vi "FPGA_Main.vi"() -> ()   [LabVIEW 2017]
uses:
  <vilib>/rvi/Emulation/niFpgaGetClockAttributes.vi
  <vilib>/rvi/Emulation/niFpgaSctlEmulationGetInTimedLoop.vi
  <vilib>/rvi/Emulation/niFpgaEmulationReportErrorSimple.vi
  <vilib>/rvi/eio/common/nirviEmuTemplateMethod_errors.vi
  <vilib>/rvi/Emulation/niFpgaCriticalErrorInLSC.vi
  <vilib>/eio/EIONode/EIONode.xnode
panel:
  out "Velocity Right (m/s)":sgl
  out "Raw ms Difference R":u32
  in  "Stop R":bool
  out "Velocity Left (m/s)":sgl
  out "Raw ms Difference L":u32
  in  "Stop L":bool
  out "BR Raw":bool
  out "BR Count":u8
  in  "Reset BR":bool
  out "BR Tape":bool
  out "FL Raw":bool
  out "FL Count":u8
  in  "Reset FL":bool
  out "BL Raw":bool
  out "BL Count":u8
  in  "Reset BL":bool
  out "BL Tape":bool
  out "FR Raw":bool
  out "FR Count":u8
  in  "Reset FR":bool
  out "Tick Count(uSec)":u32
  out "Right Velocity":sgl
  out "Left Velocity":sgl
  out "Right LS Fault":bool
  out "Left LS Fault":bool
  out "Right Tape Count":u32
  out "Left Tape Count":u32
  out "test time":u32
  out "PCS 4 Position":i16
  out "PCS 3 Position":i16
  out "PCS 2 Position":i16
  out "PCS 1 Position":i16
  out "Levitating?":bool
  out "Levitation Height":sgl format="%.14g"
  out "CJC Voltage":fxp<+/-,24,-2> format="%.26g"
  out "TC Voltages":fxp<+/-,25,-1>[](array[numeric]) format="%.26g"
  out "Reserve Battery Current":fxp<+/-,55,8>=25.777777883741592 format="%.14g"
  out "Primary Battery 2 Current":fxp<+/-,55,8>=25.777777883741592 format="%.14g"
  out "Primary Battery 1 Current":fxp<+/-,55,8>=25.777777883741592 format="%.14g"
  out "Reserve Battery Critical":bool
  out "Reserve Battery Low":bool
  out "Primary Battery 2 Critical":bool
  out "Primary Battery 2 Low":bool
  out "Primary Battery 1 Critical":bool
  out "Primary Battery 1 Low":bool
  out "Reserve Battery Voltage":sgl format="%.14g"
  out "Primary Battery 2 Voltage":sgl format="%.14g"
  out "Primary Battery 1 Voltage":sgl format="%.14g"
  out "Downstream 2 Pressure Fault":bool
  out "Ambient Pressure":sgl format="%.2f"
  out "Downstream Right Pressure":sgl format="%.2f"
  out "Tank Pressure":sgl format="%.2f"
  out "Downstream Left Pressure":sgl format="%.2f"
  out "Downstream Pressure Low":bool
  out "Tank Pressue Low":bool
  out "Downstream Pressure Fault":bool
  out "Tank Pressure Fault":bool
  out "Pusher Connected":bool
  out "IR Fault":bool
  out "IR 2 RAW":sgl format="%.21g"
  out "IR 1 RAW":sgl format="%.21g"
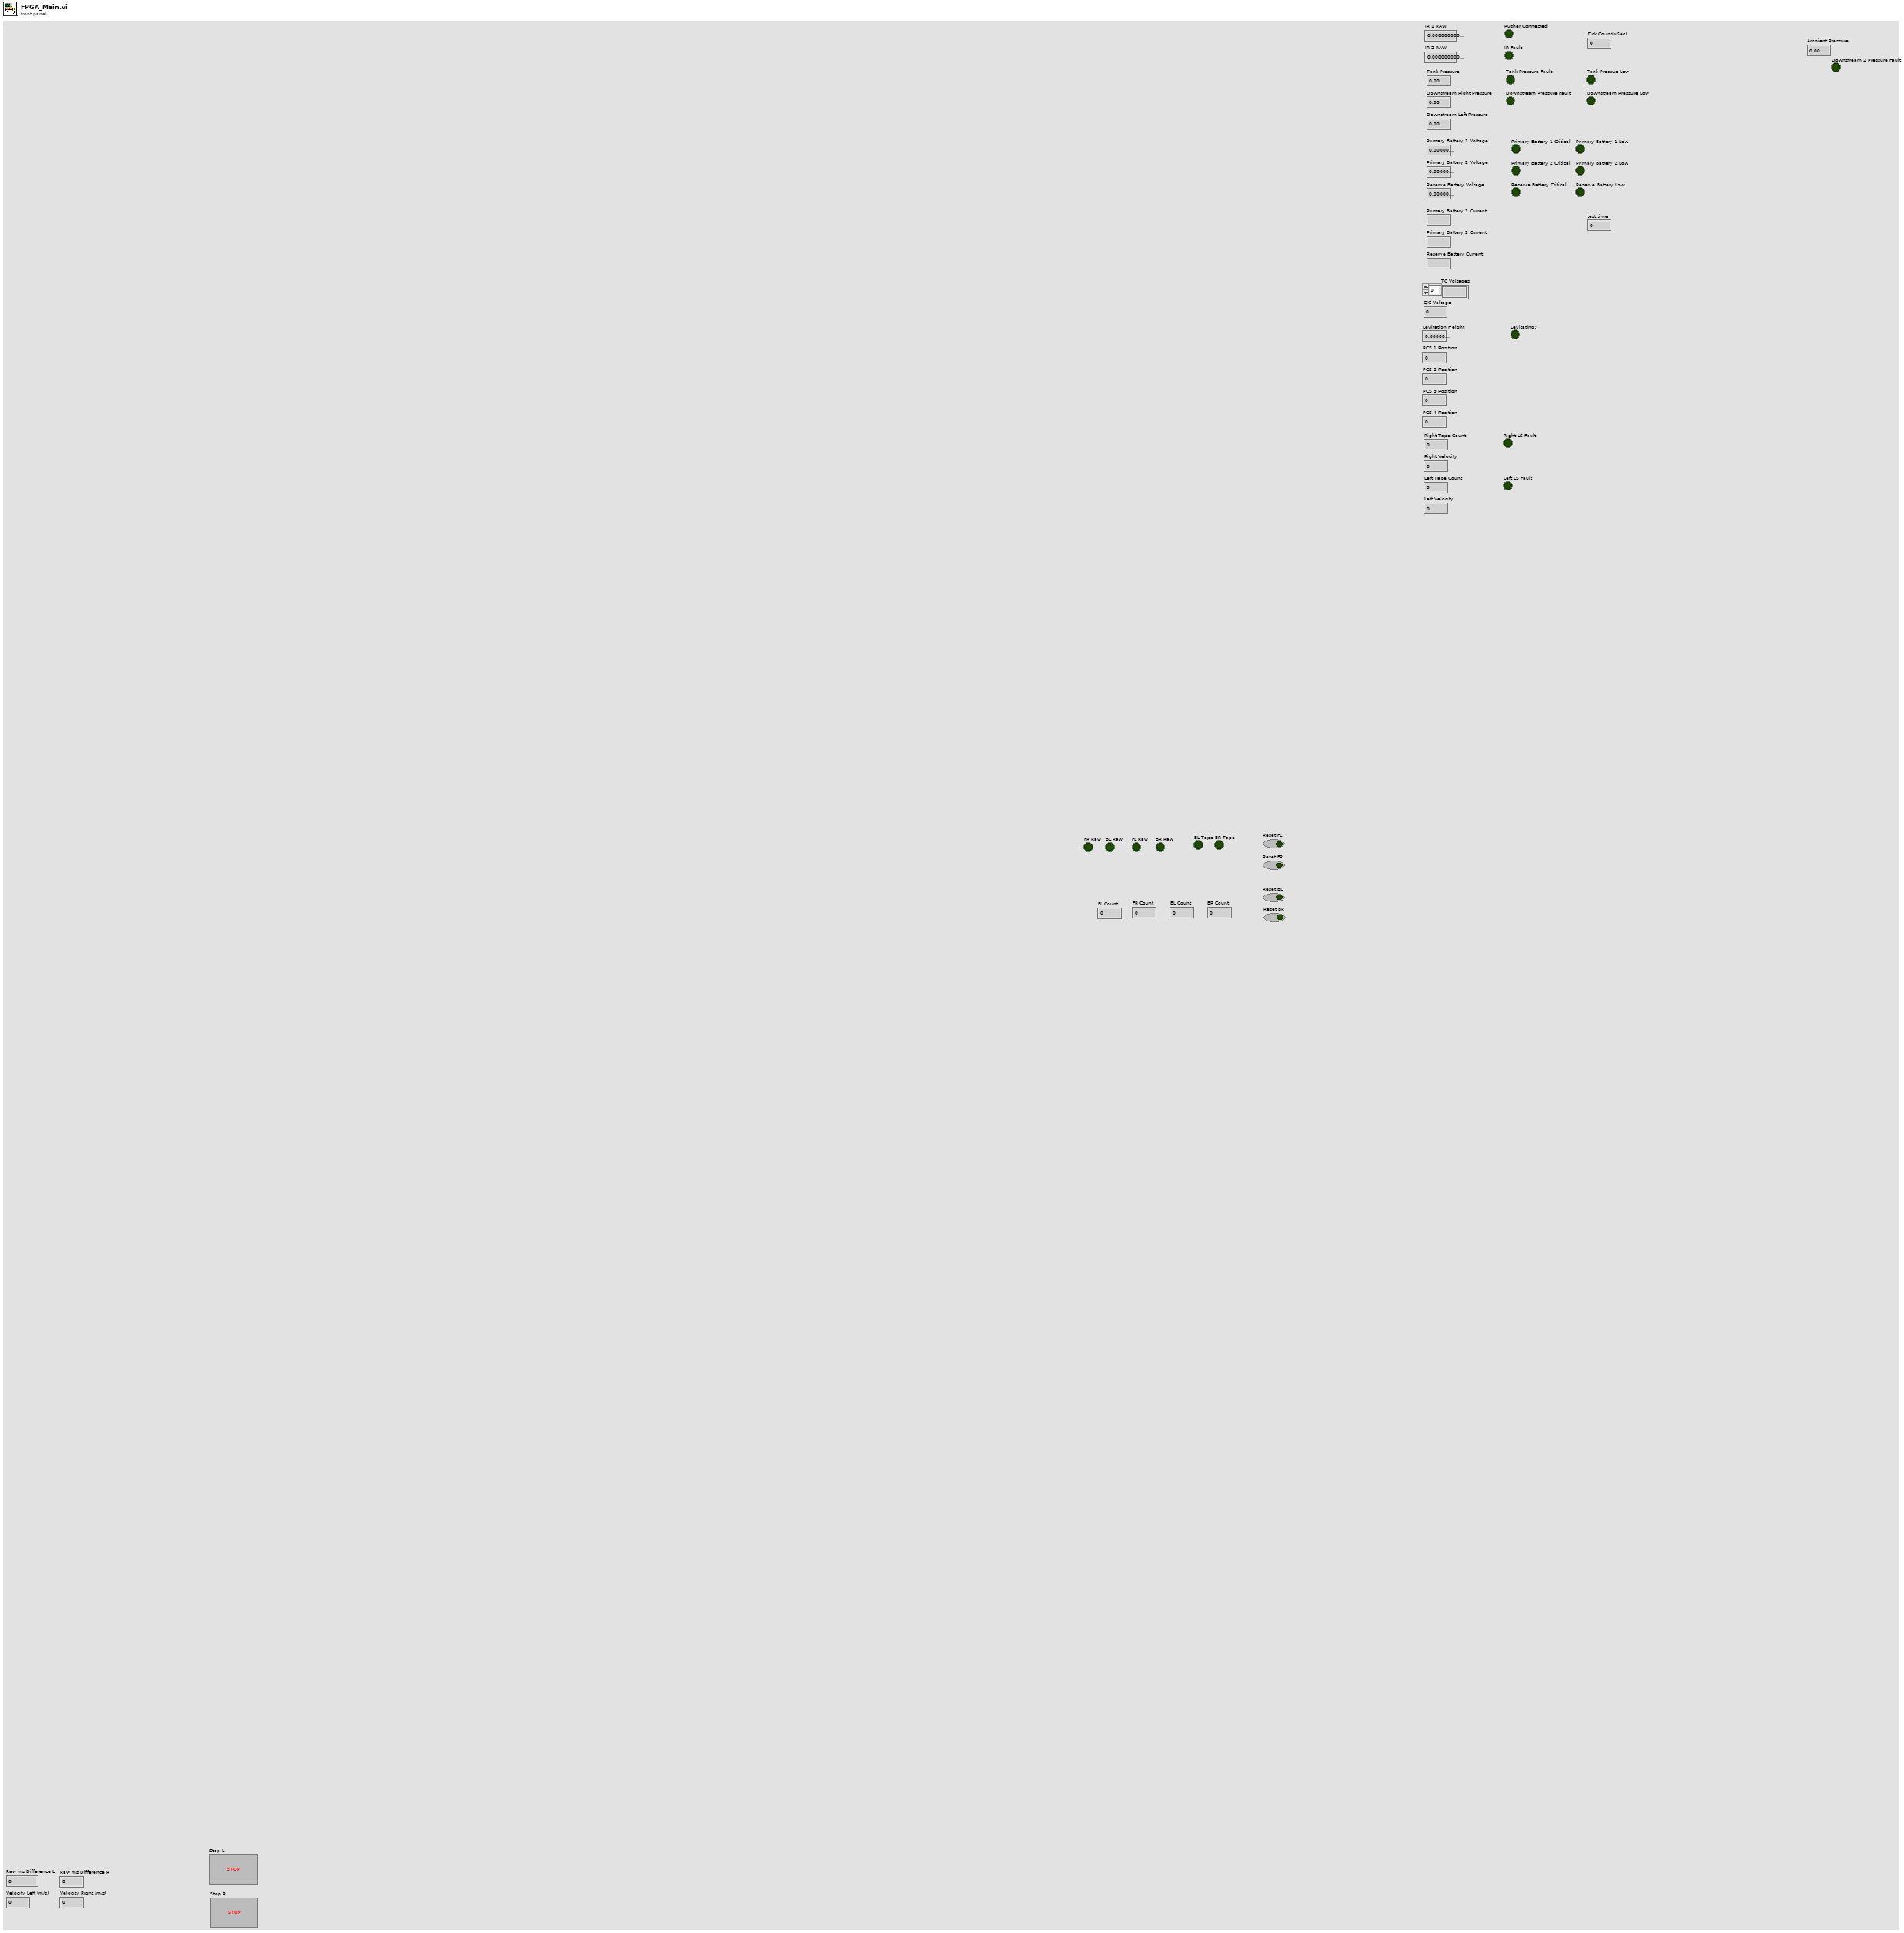
[diagram p1: front panel]
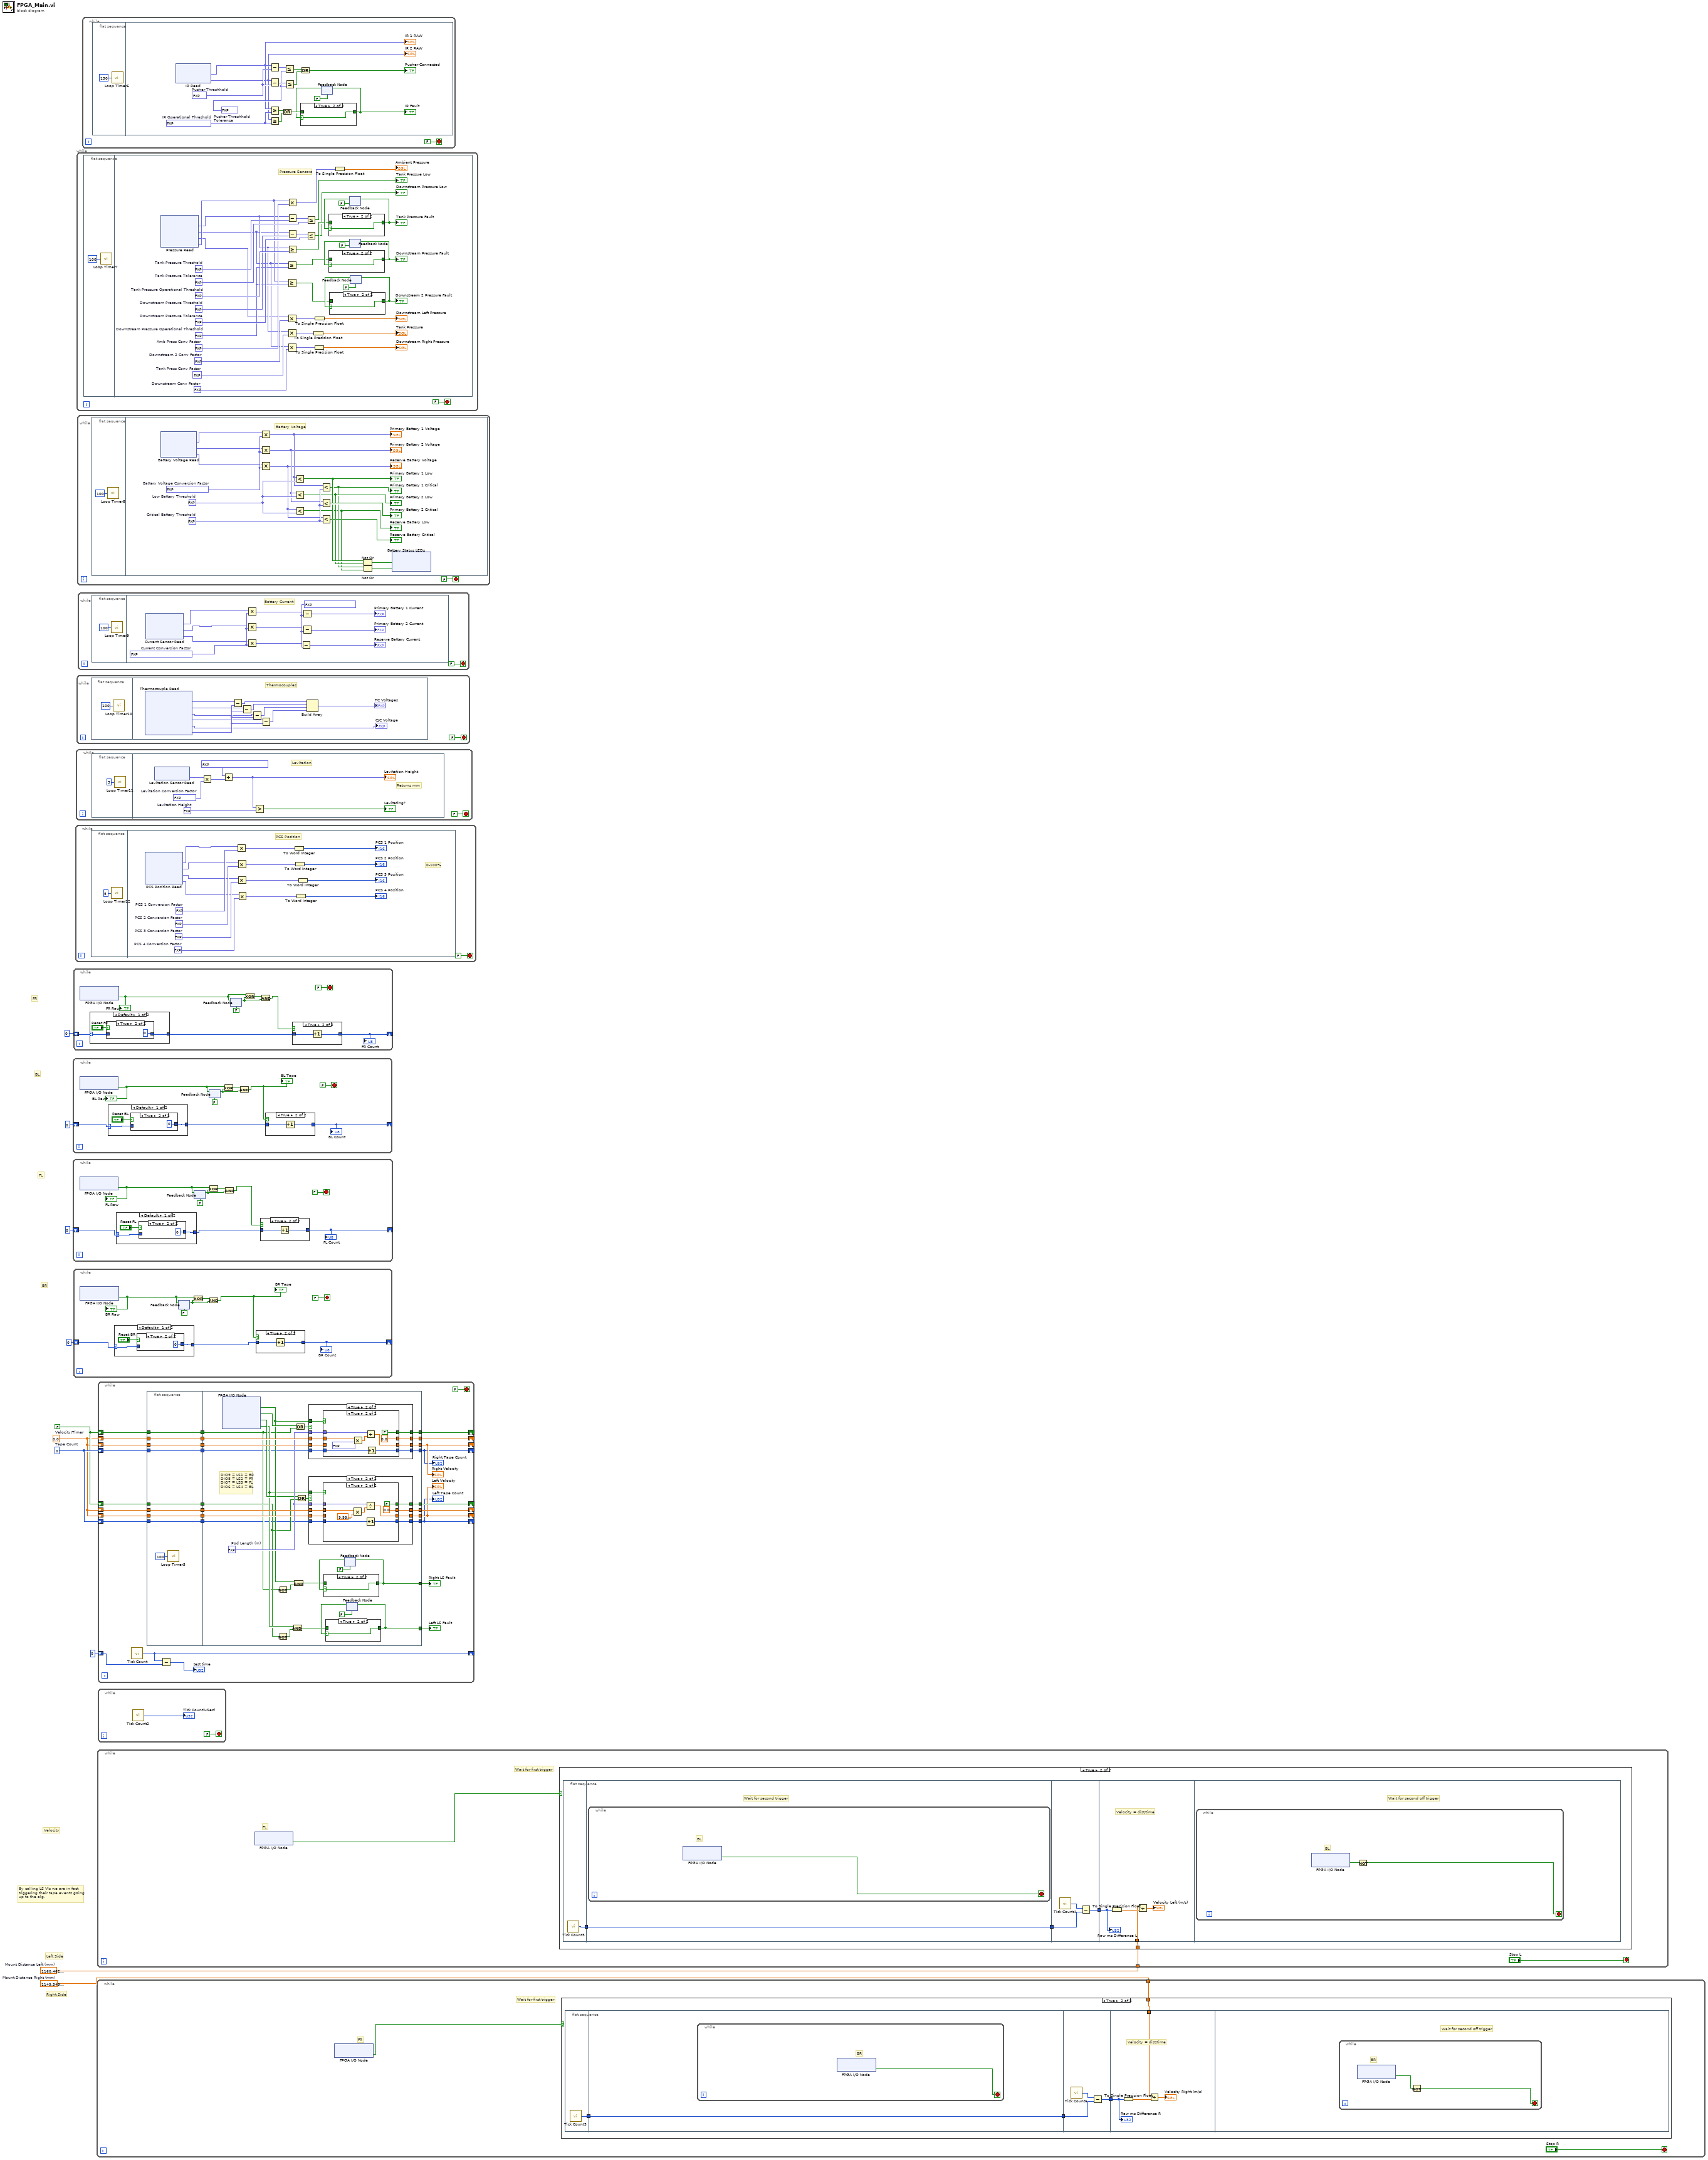
[diagram p0: block diagram]
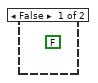
[diagram p2: hidden frame]
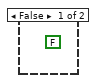
[diagram p3: hidden frame]
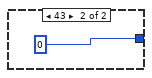
[diagram p5: hidden frame]
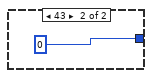
[diagram p8: hidden frame]
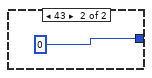
[diagram p11: hidden frame]
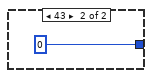
[diagram p14: hidden frame]
diagram:
  w1 = sgl 1149.35  # Mount Distance Right (mm)
  w2 = sgl 1160.4625  # Mount Distance Left (mm)
  w9 = FALSE
  w10 = u32 0  # Tape Count
  w7 = sgl 0.0  # Velocity/Timer
  # "Right Side"
  # "Left Side"
  # "By calling LS VIs we are in fact\ntriggering their tape events going\nup to the alg."
  # "Velocity"
  # "BR"
  # "FL"
  # "BL"
  # "FR"
  n1 = while {
    shift-right: [w14] -> _
    shift-left: u8 0 -> [w12]
    stop <- FALSE stop-if-true
    n2 = xnode "FPGA I/O Node"() -> ("Mod2/DIO8"=w15:bool)  [unwired: 1 in, 1 out]
    "BL Raw" <- w15
    n3 = case shown="Default" w12 {
      selector: w12 -> [w21 _]
      tunnel: [w20 u8 0] -> w11
      frame Default {
        n4 = case shown="True" "Reset BL" {
          tunnel: w21 -> [w23 _]
          tunnel: [w23 u8 0] -> w20
          frame False {
          }
          frame True {
          }
        }
      }
      frame 43 {
      }
    }
    n5 = feedback #1(FALSE ("Mod2/DIO2")) -> (w18:bool)
    n6 = feedback-in #1(w15) -> ()
    n7 = Exclusive Or(1:w18, 2:w15) -> (0:w17:bool)
    n8 = And(x=w17, y=w18) -> (x .and. y?=w13:bool)
    "BL Tape" <- w13
    n9 = case shown="True" w13 {
      tunnel: [w26 w28] -> w14
      tunnel: w11 -> [w26 w27]
      frame False {
      }
      frame True {
        n10 = Increment(x=w27) -> (x+1=w28:u8)
      }
    }
    "BL Count" <- w14
  }
  n11 = while {
    shift-right: [w31] -> _
    shift-left: u8 0 -> [w30]
    stop <- FALSE stop-if-true
    n12 = xnode "FPGA I/O Node"() -> ("Mod2/DIO7"=w33:bool)  [unwired: 1 in, 1 out]
    "FL Raw" <- w33
    n13 = case shown="Default" w30 {
      selector: w30 -> [w39 _]
      tunnel: [w38 u8 0] -> w29
      frame Default {
        n14 = case shown="True" "Reset FL" {
          tunnel: w39 -> [w41 _]
          tunnel: [w41 u8 0] -> w38
          frame False {
          }
          frame True {
          }
        }
      }
      frame 43 {
      }
    }
    n15 = feedback #2(FALSE ("Mod2/DIO2")) -> (w34:bool)
    n16 = feedback-in #2(w33) -> ()
    n17 = Exclusive Or(1:w34, 2:w33) -> (0:w35:bool)
    n18 = And(x=w35, y=w34) -> (x .and. y?=w32:bool)
    n19 = case shown="True" w32 {
      tunnel: [w44 w46] -> w31
      tunnel: w29 -> [w44 w45]
      frame False {
      }
      frame True {
        n20 = Increment(x=w45) -> (x+1=w46:u8)
      }
    }
    "FL Count" <- w31
  }
  n21 = while {
    shift-right: [w50] -> _
    shift-left: u8 0 -> [w48]
    stop <- FALSE stop-if-true
    n22 = xnode "FPGA I/O Node"() -> ("Mod2/DIO6"=w52:bool)  [unwired: 1 in, 1 out]
    "FR Raw" <- w52
    n23 = case shown="Default" w48 {
      selector: w48 -> [w57 _]
      tunnel: [w56 u8 0] -> w47
      frame Default {
        n24 = case shown="True" "Reset FR" {
          tunnel: w57 -> [w59 _]
          tunnel: [w59 u8 0] -> w56
          frame False {
          }
          frame True {
          }
        }
      }
      frame 43 {
      }
    }
    n25 = feedback #3(FALSE ("Mod2/DIO2")) -> (w53:bool)
    n26 = feedback-in #3(w52) -> ()
    n27 = Exclusive Or(1:w53, 2:w52) -> (0:w54:bool)
    n28 = And(x=w54, y=w53) -> (x .and. y?=w51:bool)
    n29 = case shown="True" w51 {
      tunnel: [w62 w64] -> w50
      tunnel: w47 -> [w62 w63]
      frame False {
      }
      frame True {
        n30 = Increment(x=w63) -> (x+1=w64:u8)
      }
    }
    "FR Count" <- w50
  }
  n31 = while {
    shift-right: [w67] -> _
    shift-left: u8 0 -> [w66]
    stop <- FALSE stop-if-true
    n32 = xnode "FPGA I/O Node"() -> ("Mod2/DIO9"=w69:bool)  [unwired: 1 in, 1 out]
    "BR Raw" <- w69
    n33 = case shown="Default" w66 {
      selector: w66 -> [w75 _]
      tunnel: [w74 u8 0] -> w65
      frame Default {
        n34 = case shown="True" "Reset BR" {
          tunnel: w75 -> [w77 _]
          tunnel: [w77 u8 0] -> w74
          frame False {
          }
          frame True {
          }
        }
      }
      frame 43 {
      }
    }
    n35 = feedback #4(FALSE ("Mod2/DIO2")) -> (w72:bool)
    n36 = feedback-in #4(w69) -> ()
    n37 = Exclusive Or(1:w72, 2:w69) -> (0:w71:bool)
    n38 = And(x=w71, y=w72) -> (x .and. y?=w68:bool)
    "BR Tape" <- w68
    n39 = case shown="True" w68 {
      tunnel: [w80 w82] -> w67
      tunnel: w65 -> [w80 w81]
      frame False {
      }
      frame True {
        n40 = Increment(x=w81) -> (x+1=w82:u8)
      }
    }
    "BR Count" <- w67
  }
  n41 = while {
    stop <- FALSE stop-if-true
    n42 = flat-sequence {
      frame #0 {
        n43 = call "Loop Timer12"("Count(mSec)"=u32 5) -> ()  [unwired: 1 out]
      }
      frame #1 {
        w97 = fxp<+,3,4> 10.0  # PCS 4 Conversion Factor
        w98 = fxp<+,3,4> 10.0  # PCS 3 Conversion Factor
        w99 = fxp<+,3,4> 10.0  # PCS 2 Conversion Factor
        w100 = fxp<+,3,4> 10.0  # PCS 1 Conversion Factor
        # "0-100%"
        # "PCS Position"
        n44 = xnode "PCS Position Read"() -> ("Mod1/AI19"=w88:fxp<+/-,24,5>, "Mod1/AI18"=w87:fxp<+/-,24,5>, "Mod1/AI17"=w86:fxp<+/-,24,5>, "Mod1/AI16"=w85:fxp<+/-,24,5>)  [unwired: 4 in, 4 out]
        n45 = Multiply(x=w88, y=w100) -> (x*y=w96:fxp<+/-,27,9>)
        n46 = Multiply(x=w87, y=w99) -> (x*y=w94:fxp<+/-,27,9>)
        n47 = Multiply(x=w86, y=w98) -> (x*y=w92:fxp<+/-,27,9>)
        n48 = Multiply(x=w85, y=w97) -> (x*y=w91:fxp<+/-,27,9>)
        n49 = To Word Integer(number=w96) -> (16bit integer=→"PCS 1 Position":i16)
        n50 = To Word Integer(number=w94) -> (16bit integer=→"PCS 2 Position":i16)
        n51 = To Word Integer(number=w91) -> (16bit integer=→"PCS 4 Position":i16)
        n52 = To Word Integer(number=w92) -> (16bit integer=→"PCS 3 Position":i16)
      }
    }
  }
  n53 = while {
    stop <- FALSE stop-if-true
    n54 = flat-sequence {
      frame #0 {
        n55 = call "Loop Timer11"("Count(mSec)"=u32 5) -> ()  [unwired: 1 out]
      }
      frame #1 {
        w106 = fxp<+,1,1> 0.0  # Levitation Height
        w109 = fxp<+/-,13,5> -9.1796875  # Levitation Conversion Factor
        # "Returns mm"
        # "Levitation"
        n56 = xnode "Levitation Sensor Read"() -> ("Mod1/AI5"=w107:fxp<+/-,24,5>)  [unwired: 1 in, 1 out]
        n57 = Multiply(x=w107, y=w109) -> (x*y=w104:fxp<+/-,36,9>)
        n58 = Add(x=fxp<+/-,36,9> 120.07999999821186 ("y"), y=w104) -> (x+y=w103:fxp<+/-,37,10>)
        "Levitation Height" <- w103
        n59 = Greater?(x=w103, y=w106) -> (0:→"Levitating?":bool)
      }
    }
  }
  n60 = while {
    stop <- FALSE stop-if-true
    n61 = flat-sequence {
      frame #0 {
        n62 = call "Loop Timer7"("Count(mSec)"=u32 100) -> ()  [unwired: 1 out]
      }
      frame #1 {
        w116 = fxp<+,7,10> 600.0  # Tank Press Conv Factor
        w117 = fxp<+,3,6> 40.0  # Downstream 2 Conv Factor
        w118 = fxp<+,2,3> 6.0  # Amb Press Conv Factor
        w143 = fxp<+/-,24,5> 1.0  # Downstream Pressure Tolerance
        w131 = fxp<+/-,24,5> 0.0  # Downstream Pressure Operational Threshold
        w144 = fxp<+/-,24,5> 1.0  # Downstream Pressure Threshold
        w146 = fxp<+/-,24,5> 1.0  # Tank Pressure Tolerance
        w145 = fxp<+/-,24,5> 1.0  # Tank Pressure Operational Threshold
        w147 = fxp<+/-,24,5> 1.0  # Tank Pressure Threshold
        w132 = fxp<+,3,6> 40.0  # Downstream Conv Factor
        # "Pressure Sensors"
        n63 = xnode "Pressure Read"() -> ("Mod1/AI1"=w114:fxp<+/-,24,5>, "Mod1/AI0"=w113:fxp<+/-,24,5>, "Mod1/AI2"=w112:fxp<+/-,24,5>, "Mod1/AI23"=w115:fxp<+/-,24,5>)  [unwired: 4 in, 4 out]
        n64 = Greater Or Equal?(x=w113, y=w131) -> (x >= y?=w135:bool)
        n65 = Greater Or Equal?(x=w115, y=w131) -> (x >= y?=w128:bool)
        n66 = Multiply(x=w112, y=w117) -> (x*y=w125:fxp<+/-,27,11>)
        n67 = Multiply(x=w114, y=w116) -> (x*y=w124:fxp<+/-,31,15>)
        n68 = Multiply(x=w113, y=w132) -> (x*y=w121:fxp<+/-,27,11>)
        n69 = Multiply(x=w115, y=w118) -> (x*y=w120:fxp<+/-,26,8>)
        n70 = Subtract(x=w114, y=w147) -> (x-y=w149:fxp<+/-,25,6>)
        n71 = Subtract(x=w113, y=w144) -> (x-y=w148:fxp<+/-,25,6>)
        n72 = Greater Or Equal?(x=w114, y=w145) -> (x >= y?=w139:bool)
        n73 = Less Or Equal?(x=w149, y=w146) -> (x <= y?=→"Tank Pressue Low":bool)
        n74 = Less Or Equal?(x=w148, y=w143) -> (x <= y?=→"Downstream Pressure Low":bool)
        n75 = To Single Precision Float(number=w124) -> (single precision float=→"Tank Pressure":sgl)
        n76 = To Single Precision Float(number=w121) -> (single precision float=→"Downstream Right Pressure":sgl)
        n77 = To Single Precision Float(number=w125) -> (single precision float=→"Downstream Left Pressure":sgl)
        n78 = To Single Precision Float(number=w120) -> (single precision float=→"Ambient Pressure":sgl)
        n79 = feedback #5(FALSE) -> (w141:bool)
        n80 = case shown="True" w141 {
          selector: w141 -> [_ w155]
          tunnel: w139 -> [w154 _]
          tunnel: [w154 w155] -> w140
          frame False {
          }
          frame True {
          }
        }
        "Tank Pressure Fault" <- w140
        n81 = feedback-in #5(w140) -> ()
        n82 = feedback #6(FALSE) -> (w137:bool)
        n83 = case shown="True" w137 {
          selector: w137 -> [_ w153]
          tunnel: w135 -> [w152 _]
          tunnel: [w152 w153] -> w136
          frame False {
          }
          frame True {
          }
        }
        "Downstream Pressure Fault" <- w136
        n84 = feedback-in #6(w136) -> ()
        n85 = feedback #7(FALSE) -> (w130:bool)
        n86 = case shown="True" w130 {
          selector: w130 -> [_ w151]
          tunnel: w128 -> [w150 _]
          tunnel: [w150 w151] -> w127
          frame False {
          }
          frame True {
          }
        }
        "Downstream 2 Pressure Fault" <- w127
        n87 = feedback-in #7(w127) -> ()
      }
    }
  }
  n88 = while {
    stop <- FALSE stop-if-true
    n89 = flat-sequence {
      frame #0 {
        n90 = call "Loop Timer10"("Count(mSec)"=u32 100) -> ()  [unwired: 1 out]
      }
      frame #1 {
        # "Thermocouples"
        n91 = xnode "Thermocouple Read"() -> ("Mod4/TC0"=w163:fxp<+/-,24,-2>, "Mod4/TC1"=w161:fxp<+/-,24,-2>, "Mod4/TC2"=w160:fxp<+/-,24,-2>, "Mod4/TC3"=w159:fxp<+/-,24,-2>, "Mod4/CJC"=→"CJC Voltage":fxp<+/-,24,-2>, "Mod4/Autozero"=w162:fxp<+/-,24,-2>)  [unwired: 6 in, 6 out]
        n92 = Subtract(x=w163, y=w162) -> (x-y=w167:fxp<+/-,25,-1>)
        n93 = Subtract(x=w161, y=w162) -> (x-y=w166:fxp<+/-,25,-1>)
        n94 = Subtract(x=w160, y=w162) -> (x-y=w165:fxp<+/-,25,-1>)
        n95 = Subtract(x=w159, y=w162) -> (x-y=w164:fxp<+/-,25,-1>)
        n96 = Build Array(w167, w166, w165, w164) -> (→"TC Voltages":fxp<+/-,25,-1>[])
      }
    }
  }
  n97 = while {
    stop <- FALSE stop-if-true
    n98 = flat-sequence {
      frame #0 {
        n99 = call "Loop Timer8"("Count(mSec)"=u32 100) -> ()  [unwired: 1 out]
      }
      frame #1 {
        w185 = fxp<+,3,5> 20.0  # Critical Battery Threshold
        w186 = fxp<+,4,5> 22.0  # Low Battery Threshold
        w187 = fxp<+,21,3> 5.651161193847656  # Battery Voltage Conversion Factor
        # "Battery Voltage"
        n100 = xnode "Battery Voltage Read"() -> ("Mod1/AI9"=w173:fxp<+/-,24,5>, "Mod1/AI7"=w172:fxp<+/-,24,5>, "Mod1/AI6"=w171:fxp<+/-,24,5>)  [unwired: 3 in, 3 out]
        n101 = Multiply(x=w173, y=w187) -> (x*y=w176:fxp<+/-,45,8>)
        "Primary Battery 1 Voltage" <- w176
        n102 = Multiply(x=w172, y=w187) -> (x*y=w175:fxp<+/-,45,8>)
        "Primary Battery 2 Voltage" <- w175
        n103 = Multiply(x=w171, y=w187) -> (x*y=w174:fxp<+/-,45,8>)
        "Reserve Battery Voltage" <- w174
        n104 = Less?(x=w176, y=w186) -> (x < y?=w180:bool)
        "Primary Battery 1 Low" <- w180
        n105 = Less?(x=w175, y=w186) -> (x < y?=w179:bool)
        "Primary Battery 2 Low" <- w179
        n106 = Less?(x=w174, y=w186) -> (x < y?=w177:bool)
        "Reserve Battery Low" <- w177
        n107 = Less?(x=w176, y=w185) -> (x < y?=w178:bool)
        "Primary Battery 1 Critical" <- w178
        n108 = Less?(x=w175, y=w185) -> (x < y?=→"Primary Battery 2 Critical":bool)
        n109 = Less?(x=w174, y=w185) -> (x < y?=→"Reserve Battery Critical":bool)
        n110 = Not Or(1:w179, 2:w180) -> (0:w181:bool)
        n111 = Not Or(1:w177, 2:w178) -> (0:w182:bool)
        n112 = xnode "Battery Status LEDs"("Mod2/DIO0"=w181, "Mod2/DIO1"=w182) -> ()  [unwired: 2 in, 2 out]
      }
    }
  }
  n113 = while {
    stop <- FALSE stop-if-true
    n114 = flat-sequence {
      frame #0 {
        n115 = call "Loop Timer9"("Count(mSec)"=u32 100) -> ()  [unwired: 1 out]
      }
      frame #1 {
        w199 = fxp<+,43,2> 2.6666665077209473
        w200 = fxp<+,31,3> 5.33333332836628  # Current Conversion Factor
        # "Battery Current"
        n116 = xnode "Current Sensor Read"() -> ("Mod1/AI13"=w192:fxp<+/-,24,5>, "Mod1/AI12"=w191:fxp<+/-,24,5>, "Mod1/AI10"=w190:fxp<+/-,24,5>)  [unwired: 3 in, 3 out]
        n117 = Multiply(x=w192, y=w200) -> (x*y=w197:fxp<+/-,55,8>)
        n118 = Multiply(x=w191, y=w200) -> (x*y=w196:fxp<+/-,55,8>)
        n119 = Multiply(x=w190, y=w200) -> (x*y=w195:fxp<+/-,55,8>)
        n120 = Subtract(x=w195, y=w199) -> (x-y=→"Reserve Battery Current":fxp<+/-,55,8>)
        n121 = Subtract(x=w197, y=w199) -> (x-y=→"Primary Battery 1 Current":fxp<+/-,55,8>)
        n122 = Subtract(x=w196, y=w199) -> (x-y=→"Primary Battery 2 Current":fxp<+/-,55,8>)
      }
    }
  }
  n123 = while {
    stop <- FALSE stop-if-true
    n124 = flat-sequence {
      frame #0 {
        n125 = call "Loop Timer6"("Count(mSec)"=u32 150) -> ()  [unwired: 1 out]
      }
      frame #1 {
        w207 = fxp<+,7,2> 3.1875  # Pusher Threshhold
        w206 = fxp<+,6,1> 1.09375  # Pusher Threshhold Tolerance
        w205 = fxp<+,21,3> 4.200000762939453  # IR Operational Threshold
        n126 = xnode "IR Read"() -> ("Mod1/AI3"=w204:fxp<+/-,24,5>, "Mod1/AI4"=w203:fxp<+/-,24,5>)  [unwired: 2 in, 2 out]
        "IR 1 RAW" <- w204
        "IR 2 RAW" <- w203
        n127 = Subtract(x=w204, y=w207) -> (x-y=w218:fxp<+/-,25,6>)
        n128 = Subtract(x=w203, y=w207) -> (x-y=w217:fxp<+/-,25,6>)
        n129 = Greater Or Equal?(x=w204, y=w205) -> (x >= y?=w214:bool)
        n130 = Greater Or Equal?(x=w203, y=w205) -> (x >= y?=w213:bool)
        n131 = Or(x=w214, y=w213) -> (x .or. y?=w210:bool)
        n132 = Less Or Equal?(x=w218, y=w206) -> (x <= y?=w216:bool)
        n133 = Less Or Equal?(x=w217, y=w206) -> (x <= y?=w215:bool)
        n134 = Or(x=w216, y=w215) -> (x .or. y?=→"Pusher Connected":bool)
        n135 = feedback #8(FALSE) -> (w209:bool)
        n136 = case shown="True" w209 {
          selector: w209 -> [_ w220]
          tunnel: w210 -> [w219 _]
          tunnel: [w219 w220] -> w208
          frame False {
          }
          frame True {
          }
        }
        "IR Fault" <- w208
        n137 = feedback-in #8(w208) -> ()
      }
    }
  }
  n138 = while {
    tunnel: w1 -> [w222]
    stop <- "Stop R" stop-if-true
    # "FR"
    # "Wait for first trigger"
    n139 = xnode "FPGA I/O Node"() -> ("Mod2/DIO6"=w221:bool)  [unwired: 1 in, 1 out]
    n140 = case shown="True" w221 {
      tunnel: w222 -> [_ w224]
      frame False {
        (unwired) FALSE
      }
      frame True {
        n141 = flat-sequence {
          tunnel: [w228] -> w227
          tunnel: w227 -> [w229]
          tunnel: [w229] -> w226
          tunnel: w226 -> [w232]
          tunnel: [w231] -> w225
          tunnel: w225 -> [w237]
          tunnel: w224 -> [w235]
          frame #0 {
            n142 = call "Tick Count5"() -> ("Tick Count(mSec)"=w228:u32)
          }
          frame #1 {
            n143 = while {
              stop <- w230 stop-if-true
              # "BR"
              n144 = xnode "FPGA I/O Node"() -> ("Mod2/DIO9"=w230:bool)  [unwired: 1 in, 1 out]
            }
          }
          frame #2 {
            n145 = call "Tick Count6"() -> ("Tick Count(mSec)"=w233:u32)
            n146 = Subtract(x=w233, y=w232) -> (x-y=w231:u32)
          }
          frame #3 {
            # "Velocity = dist/time"
            n147 = To Single Precision Float(number=w237) -> (single precision float=w236:sgl)
            n148 = Divide(x=w235, y=w236) -> (x/y=→"Velocity Right (m/s)":sgl)
            "Raw ms Difference R" <- w237
          }
          frame #4 {
            # "Wait for second off trigger"
            n149 = while {
              stop <- w238 stop-if-true
              # "BR"
              n150 = xnode "FPGA I/O Node"() -> ("Mod2/DIO9"=w239:bool)  [unwired: 1 in, 1 out]
              n151 = Not(x=w239) -> (.not. x?=w238:bool)
            }
          }
        }
      }
    }
  }
  n152 = while {
    tunnel: w2 -> [w241]
    stop <- "Stop L" stop-if-true
    # "FL"
    # "Wait for first trigger"
    n153 = xnode "FPGA I/O Node"() -> ("Mod2/DIO7"=w240:bool)  [unwired: 1 in, 1 out]
    n154 = case shown="True" w240 {
      tunnel: w241 -> [_ w243]
      frame False {
        (unwired) FALSE
      }
      frame True {
        n155 = flat-sequence {
          tunnel: [w247] -> w246
          tunnel: w246 -> [w248]
          tunnel: [w248] -> w245
          tunnel: w245 -> [w251]
          tunnel: [w250] -> w244
          tunnel: w244 -> [w255]
          tunnel: w243 -> [w253]
          frame #0 {
            n156 = call "Tick Count3"() -> ("Tick Count(mSec)"=w247:u32)
          }
          frame #1 {
            # "Wait for second trigger"
            n157 = while {
              stop <- w249 stop-if-true
              # "BL"
              n158 = xnode "FPGA I/O Node"() -> ("Mod2/DIO8"=w249:bool)  [unwired: 1 in, 1 out]
            }
          }
          frame #2 {
            n159 = call "Tick Count4"() -> ("Tick Count(mSec)"=w252:u32)
            n160 = Subtract(x=w252, y=w251) -> (x-y=w250:u32)
          }
          frame #3 {
            # "Velocity = dist/time"
            n161 = To Single Precision Float(number=w255) -> (single precision float=w254:sgl)
            n162 = Divide(x=w253, y=w254) -> (x/y=→"Velocity Left (m/s)":sgl)
            "Raw ms Difference L" <- w255
          }
          frame #4 {
            # "Wait for second off trigger"
            n163 = while {
              stop <- w257 stop-if-true
              # "BL"
              n164 = xnode "FPGA I/O Node"() -> ("Mod2/DIO8"=w258:bool)  [unwired: 1 in, 1 out]
              n165 = Not(x=w258) -> (.not. x?=w257:bool)
            }
          }
        }
      }
    }
  }
  n166 = while {
    shift-right: [w288] -> _
    shift-left: w9 -> [w277]
    shift-right: [w287] -> _
    shift-left: w9 -> [w280]
    shift-right: [w285] -> _
    shift-left: w7 -> [w286]
    shift-right: [w282] -> _
    shift-left: w7 -> [w284]
    shift-right: [w281] -> _
    shift-left: w7 -> [w283]
    shift-right: [w274] -> _
    shift-left: w10 -> [w275]
    shift-right: [w272] -> _
    shift-left: w10 -> [w273]
    shift-right: [w263] -> _
    shift-left: u32 0 ("Tick Count(uSec)") -> [w262]
    shift-right: [w259] -> _
    shift-left: w7 -> [w260]
    stop <- FALSE stop-if-true
    n167 = call "Tick Count"() -> ("Tick Count(uSec)"=w263:u32)
    n168 = flat-sequence {
      tunnel: w273 -> [w290]
      tunnel: w275 -> [w291]
      tunnel: w277 -> [w292]
      tunnel: w280 -> [w293]
      tunnel: w283 -> [w294]
      tunnel: w284 -> [w295]
      tunnel: w286 -> [w296]
      tunnel: w260 -> [w297]
      tunnel: [w297] -> w271
      tunnel: [w296] -> w270
      tunnel: [w295] -> w269
      tunnel: [w294] -> w268
      tunnel: [w293] -> w267
      tunnel: [w292] -> w266
      tunnel: [w291] -> w265
      tunnel: [w290] -> w264
      tunnel: [w327] -> w288
      tunnel: [w326] -> w287
      tunnel: [w325] -> w259
      tunnel: [w322] -> w285
      tunnel: [w318] -> w282
      tunnel: [w317] -> w281
      tunnel: [w308] -> w279
      tunnel: [w304] -> w278
      tunnel: [w300] -> w274
      tunnel: [w298] -> w272
      tunnel: w271 -> [w324]
      tunnel: w270 -> [w323]
      tunnel: w269 -> [w320]
      tunnel: w268 -> [w319]
      tunnel: w267 -> [w311]
      tunnel: w266 -> [w302]
      tunnel: w265 -> [w301]
      tunnel: w264 -> [w299]
      frame #0 {
        n169 = call "Loop Timer5"("Count(uSec)"=u32 100) -> ()  [unwired: 1 out]
      }
      frame #1 {
        w321 = fxp<+,1,1> 0.0  # Pod Length (m)
        # "DIO9 = LS1 = BR\nDIO8 = LS2 = FR\nDIO7 = LS3 = FL\nDIO6 = LS4 = BL"
        n170 = xnode "FPGA I/O Node"() -> ("Mod2/DIO9"=w316:bool, "Mod2/DIO6"=w328:bool, "Mod2/DIO7"=w313:bool, "Mod2/DIO8"=w312:bool)  [unwired: 4 in, 4 out]
        n171 = Not(x=w302) -> (.not. x?=w315:bool)
        n172 = Not(x=w311) -> (.not. x?=w314:bool)
        n173 = And(x=w312, y=w314) -> (x .and. y?=w303:bool)
        n174 = And(x=w316, y=w315) -> (x .and. y?=w307:bool)
        n175 = Or(x=w328, y=w302) -> (x .or. y?=w330:bool)
        n176 = Or(x=w313, y=w311) -> (x .or. y?=w329:bool)
        n177 = case shown="True" w330 {
          selector: w330 -> [w363 _]
          tunnel: w316 -> [_ w374]
          tunnel: [w363 w373] -> w327
          tunnel: [w364 w372] -> w325
          tunnel: w324 -> [w364 w371]
          tunnel: w321 -> [_ w370]
          tunnel: [w365 w369] -> w318
          tunnel: w320 -> [w365 w368]
          tunnel: w301 -> [w362 w367]
          tunnel: [w362 w366] -> w300
          frame False {
          }
          frame True {
            n178 = case shown="True" w374 {
              tunnel: [TRUE FALSE] -> w373
              tunnel: [w377 sgl 0.0] -> w372
              tunnel: w371 -> [w378 w380]
              tunnel: w370 -> [_ w388]
              tunnel: [w376 w387] -> w369
              tunnel: w368 -> [w376 _]
              tunnel: w367 -> [w375 w382]
              tunnel: [w375 w381] -> w366
              frame False {
                n179 = Increment(x=w378) -> (x+1=w377:sgl)
              }
              frame True {
                n180 = Multiply(x=w380, y=fxp<+,5,-13> 9.918212890625e-05) -> (x*y=w383:sgl)
                n181 = Divide(x=w388, y=w383) -> (x/y=w387:sgl)
                n182 = Increment(x=w382) -> (x+1=w381:u32)
              }
            }
          }
        }
        n183 = case shown="True" w329 {
          selector: w329 -> [w336 _]
          tunnel: w312 -> [_ w347]
          tunnel: [w336 w346] -> w326
          tunnel: w323 -> [w337 w345]
          tunnel: [w337 w344] -> w322
          tunnel: w321 -> [_ w343]
          tunnel: [w338 w342] -> w317
          tunnel: w319 -> [w338 w341]
          tunnel: w299 -> [w335 w340]
          tunnel: [w335 w339] -> w298
          frame False {
          }
          frame True {
            n184 = case shown="True" w347 {
              tunnel: [TRUE FALSE] -> w346
              tunnel: w345 -> [w350 w353]
              tunnel: [w351 sgl 0.0] -> w344
              tunnel: w343 -> [_ w357]
              tunnel: [w349 w356] -> w342
              tunnel: w341 -> [w349 _]
              tunnel: w340 -> [w348 w355]
              tunnel: [w348 w354] -> w339
              frame False {
                n185 = Increment(x=w350) -> (x+1=w351:sgl)
              }
              frame True {
                n186 = Multiply(x=w353, y=sgl 0.0001) -> (x*y=w358:sgl)
                n187 = Divide(x=w357, y=w358) -> (x/y=w356:sgl)
                n188 = Increment(x=w355) -> (x+1=w354:u32)
              }
            }
          }
        }
        n189 = feedback #9(FALSE) -> (w309:bool)
        n190 = case shown="True" w309 {
          selector: w309 -> [_ w334]
          tunnel: w307 -> [w333 _]
          tunnel: [w333 w334] -> w308
          frame False {
          }
          frame True {
          }
        }
        n191 = feedback-in #9(w308) -> ()
        n192 = feedback #10(FALSE) -> (w305:bool)
        n193 = case shown="True" w305 {
          selector: w305 -> [_ w332]
          tunnel: w303 -> [w331 _]
          tunnel: [w331 w332] -> w304
          frame False {
          }
          frame True {
          }
        }
        n194 = feedback-in #10(w304) -> ()
      }
    }
    n195 = Subtract(x=w263, y=w262) -> (x-y=→"test time":u32)
    "Right Velocity" <- w282
    "Left Velocity" <- w281
    "Right LS Fault" <- w279
    "Left LS Fault" <- w278
    "Right Tape Count" <- w274
    "Left Tape Count" <- w272
  }
  n196 = while {
    stop <- FALSE stop-if-true
    n197 = call "Tick Count2"() -> ("Tick Count(uSec)"=→"Tick Count(uSec)":u32)
  }
